vi "Error to System Log.vi"(8 "error in (no error)":errorcluster, 9 "Previous State":string, 11 "Clear?":bool) -> (0 "error out":errorcluster, 3 "Log Message":string)   [LabVIEW 2011]
doc: "Sends error details to the system log.\n\n\nVersion 1.1 - 6/1/2010\n\nPhaeron, Inc.\nwww.phaeron.com\ninfo@phaeron.com"
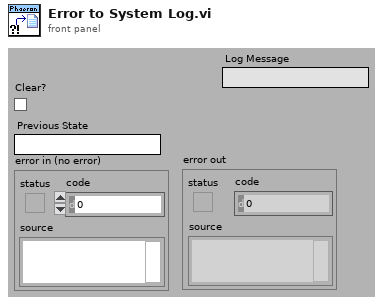
[diagram p1: front panel]
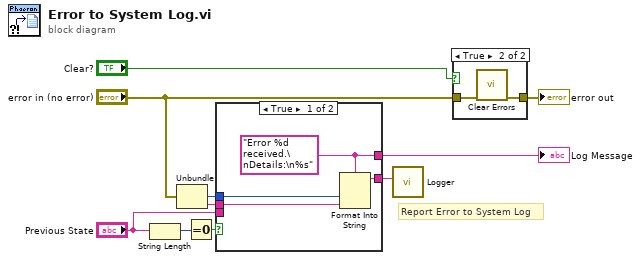
[diagram p0: block diagram]
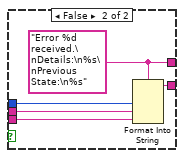
[diagram p2: hidden frame]
diagram:
  # "Report Error to System Log"
  n1 = String Length(string="Previous State") -> (length=w3:i32)
  n2 = Unbundle("error in (no error)") -> ("code"=w8:i32, "source"=w9:string)  [unwired: 1 out]
  n3 = Equal To 0?(x=w3) -> (x = 0?=w2:bool)
  n4 = case shown="True" w2 {
    tunnel: [w14 w19] -> w10
    tunnel: w9 -> [w13 w18]
    tunnel: w8 -> [w12 w17]
    tunnel: [w11 w16] -> w7
    tunnel: "Previous State" -> [_ w15]
    frame True {
      w11 = "Error %d received.\nDetails:\n%s"
      n5 = Format Into String(format string=w11, w12, w13) -> (resulting string=w14:string)  [unwired: 2 in, 1 out]
    }
    frame False {
      w16 = "Error %d received.\nDetails:\n%s\nPrevious State:\n%s"
      n6 = Format Into String(format string=w16, w17, w18, w15) -> (resulting string=w19:string)  [unwired: 2 in, 1 out]
    }
  }
  "Log Message" <- w7
  n7 = call "Logger.vi"("Information"=w10) -> ()  [unwired: 7 in, 4 out]
  n8 = case shown="True" "Clear?" {
    tunnel: "error in (no error)" -> [w20 w22]
    tunnel: [w20 w21] -> w5
    frame False {
    }
    frame True {
      n9 = call <vilib>:"Clear Errors.vi"("error in (no error)"=w22) -> ("error out"=w21:errorcluster)  [unwired: 6 in]
    }
  }
  "error out" <- w5
